vi "AWS Process Output.vi"(8 "error in":errorcluster, 10 "standard output":string, 11 "LV-Data.AWS CLI":refnum<class "LV-Data.AWS CLI.lvclass">) -> (0 "error out":errorcluster, 1 "Array Output":string[](array[string]), 2 "standard output":string, 3 "LV-Data.AWS CLI out":refnum<class "LV-Data.AWS CLI.lvclass">)   [LabVIEW 2019, in "LV-Data.AWS CLI.lvclass"]
uses:
  LV-Data.AWS CLI.lvclass
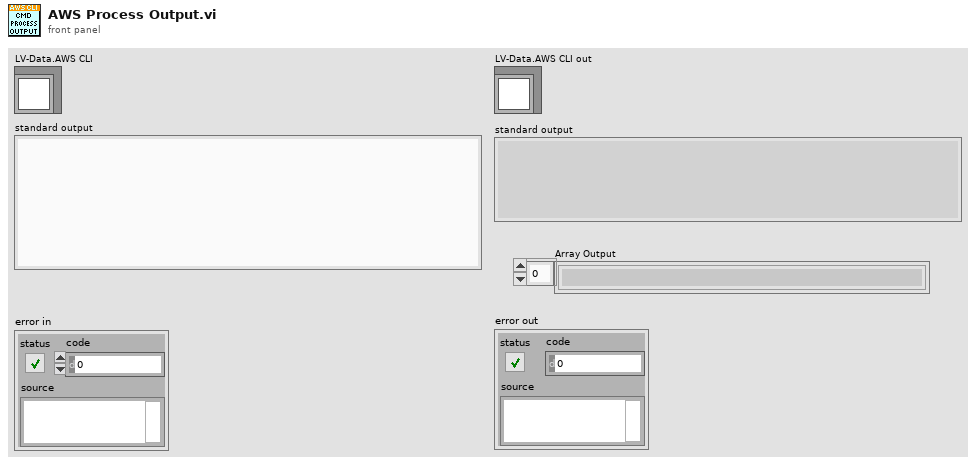
[diagram p1: front panel]
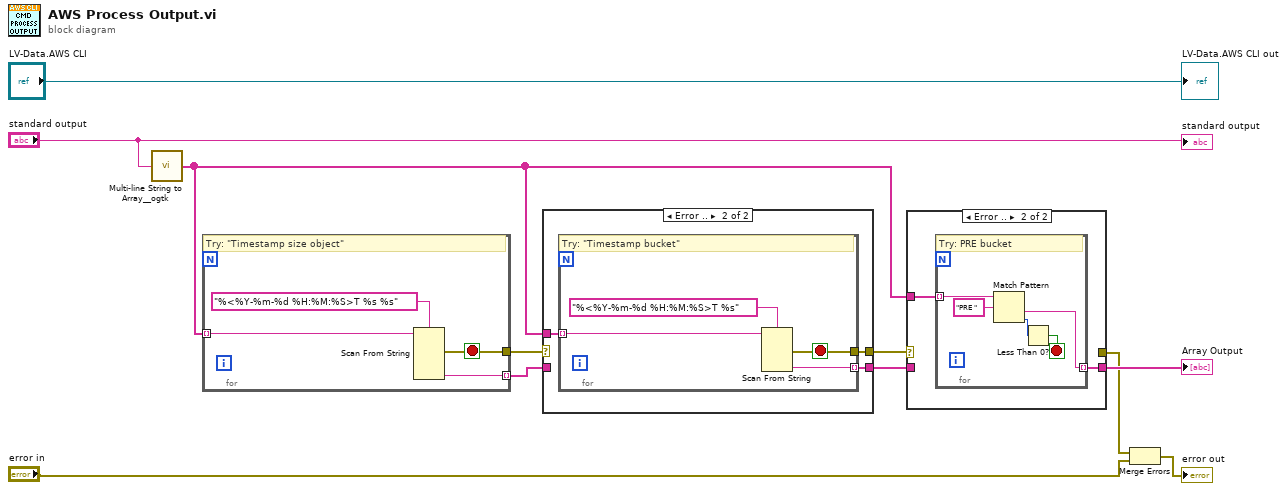
[diagram p0: block diagram]
diagram:
  n1 = call <userlib>:"Multi-line String to Array__ogtk.vi"("string"="standard output") -> ("lines"=w4:string[])
  n2 = for {
    tunnel: w4 -> [w15] mode=indexing
    tunnel: [w13] -> w3
    tunnel: [w12] -> w2 mode=indexing
    stop <- w13 stop-if-true
    # "Try: \"Timestamp size object\""
    n3 = Scan From String(format string="%<%Y-%m-%d %H:%M:%S>T %s %s", input string=w15) -> (error out=w13:errorcluster, output 3=w12:string)  [unwired: 7 in, 2 out]
  }
  n4 = case shown="Error .." w3 {
    selector: w3 -> [w17 _]
    tunnel: [w17 w20] -> w10
    tunnel: [w16 w19] -> w9
    tunnel: w4 -> [_ w18]
    tunnel: w2 -> [w16 _]
    frame No Error {
    }
    frame Error {
      n5 = for {
        tunnel: w18 -> [w24] mode=indexing
        tunnel: [w22] -> w20
        tunnel: [w21] -> w19 mode=indexing
        stop <- w22 stop-if-true
        # "Try: \"Timestamp bucket\""
        n6 = Scan From String(format string="%<%Y-%m-%d %H:%M:%S>T %s", input string=w24) -> (error out=w22:errorcluster, output 2=w21:string)  [unwired: 5 in, 2 out]
      }
    }
  }
  n7 = case shown="Error .." w10 {
    selector: w10 -> [w25 _]
    tunnel: w4 -> [_ w28]
    tunnel: w9 -> [w26 _]
    tunnel: [w26 w27] -> w8
    tunnel: [w25 _] -> w1
    frame No Error {
    }
    frame Error {
      n8 = for {
        tunnel: w28 -> [w33] mode=indexing
        tunnel: [w31] -> w27 mode=indexing
        stop <- w29 stop-if-true
        # "Try: PRE bucket"
        n9 = Match Pattern(string=w33, regular expression="PRE ") -> (after substring=w31:string, offset past match=w30:i32)  [unwired: 1 in, 2 out]
        n10 = Less Than 0?(x=w30) -> (x < 0?=w29:bool)
      }
    }
  }
  "Array Output" <- w8
  n11 = Merge Errors(w1, "error in") -> (→"error out":errorcluster)
  "standard output" <- "standard output"
  "LV-Data.AWS CLI out" <- "LV-Data.AWS CLI"
